vi "ABOUT.vi"   [LabVIEW 2020]
panel:
  # "Custom Device Configurator\n\nDeveloped by Felipe Flores at National Intruments 2020 \n\nThis is a total free example project. This code is not supported by National Instruments\nby any means."
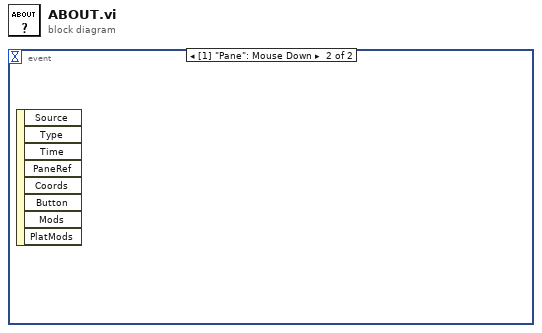
[diagram p0: block diagram]
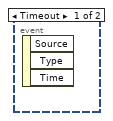
[diagram p2: hidden frame]
diagram:
  n1 = event shown="[1] \"Pane\": Mouse Down" {
    selector: _ -> [_ _]
    dyn-events: _ -> [_ _]
    timeout: _ -> [_ _]
    event Timeout {
      n2 = event-data() -> ()  [unwired: 1 in, 3 out]
    }
    event Mouse Down {
      n3 = event-data() -> ()  [unwired: 1 in, 8 out]
    }
  }
